vi "FollowBeeCircle.vi"(0 "Way Point X":dbl, 1 "Way Point Y":dbl, 2 "X Pos":dbl, 3 "Y Pos":dbl, 4 "Heading":dbl) -> (5 "Rudder Angle":dbl)   [LabVIEW 2014]
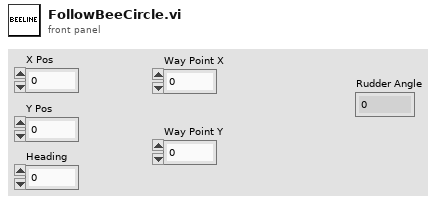
[diagram p1: front panel]
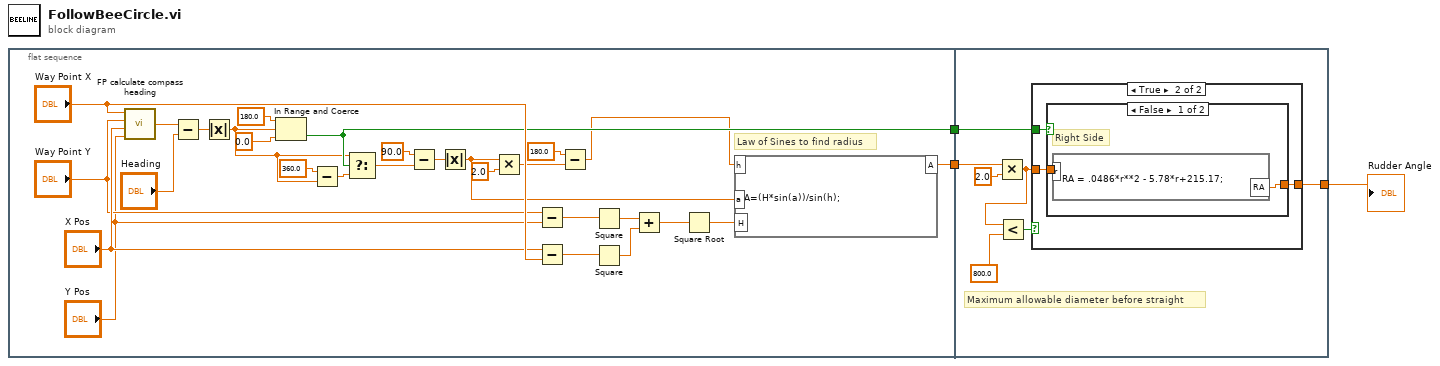
[diagram p0: block diagram]
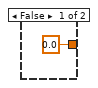
[diagram p2: hidden frame]
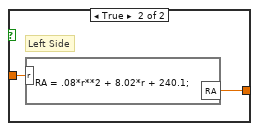
[diagram p3: hidden frame]
diagram:
  n1 = flat-sequence {
    tunnel: [w18] -> w3
    tunnel: [w7] -> w1
    tunnel: w3 -> [w38]
    tunnel: [w35] -> w2
    tunnel: w1 -> [w37]
    frame #0 {
      # "Law of Sines to find radius"
      n2 = call "FP calculate compass heading.vi"("Y Location"="Y Pos", "X Location"="X Pos", "Waypoint Y"="Way Point Y", "Waypoint X"="Way Point X") -> ("Heading"=w31:dbl)
      n3 = Subtract(x=w31, y="Heading") -> (x-y=w6:dbl)
      n4 = Absolute Value(x=w6) -> (abs(x)=w4:dbl)
      n5 = In Range and Coerce(upper limit=180.0, x=w4, lower limit=0.0) -> (In Range?=w18:bool)  [unwired: 1 out]
      n6 = Subtract(x=360.0 ("upper limit"), y=w4) -> (x-y=w5:dbl)
      n7 = Select(t=w4, s=w18, f=w5) -> (s? t:f=w15:dbl)
      n8 = Subtract(x=90.0 ("upper limit"), y=w15) -> (x-y=w14:dbl)
      n9 = Absolute Value(x=w14) -> (abs(x)=w10:dbl)
      n10 = Multiply(x=w10, y=2.0) -> (x*y=w11:dbl)
      n11 = Subtract(x="Way Point Y", y="Y Pos") -> (x-y=w23:dbl)
      n12 = Subtract(x="X Pos", y="Way Point X") -> (x-y=w22:dbl)
      n13 = Subtract(x=180.0 ("upper limit"), y=w11) -> (x-y=w8:dbl)
      n14 = Square(x=w23) -> (x^2=w20:dbl)
      n15 = Square(x=w22) -> (x^2=w21:dbl)
      n16 = Add(x=w20, y=w21) -> (x+y=w19:dbl)
      n17 = Square Root(x=w19) -> (sqrt(x)=w9:dbl)
      n18 = formula code="A=(H*sin(a))/sin(h);"("a"=w10, "H"=w9, "h"=w8) -> ("A"=w7:dbl)
    }
    frame #1 {
      # "Maximum allowable diameter before straight"
      n19 = Multiply(x=w37, y=2.0) -> (x*y=w34:dbl)
      n20 = Less?(x=w34, y=800.0) -> (x < y?=w32:bool)
      n21 = case shown="True" w32 {
        tunnel: w38 -> [_ w42]
        tunnel: [0.0 ("RA") w41] -> w35
        tunnel: w34 -> [_ w40]
        frame False {
        }
        frame True {
          n22 = case shown="False" w42 {
            tunnel: w40 -> [w44 w46]
            tunnel: [w43 w45] -> w41
            frame False {
              # "Right Side"
              n23 = formula code="RA = .0486*r**2 - 5.78*r+215.17;"("r"=w44) -> ("RA"=w43:dbl)
            }
            frame True {
              # "Left Side"
              n24 = formula code="RA = .08*r**2 + 8.02*r + 240.1;"("r"=w46) -> ("RA"=w45:dbl)
            }
          }
        }
      }
    }
  }
  "Rudder Angle" <- w2
